vi "Clear-value-reference.vi"(8 "error in (no error)":errorcluster, 11 "Correct. params. ref.":refnum<data-value>) -> (0 "error out":errorcluster, 3 "Correct params out":refnum<class "CV-Correction.lvclass">)   [LabVIEW 2013, in "CameraVision.lvlib" / "CV-Correction.lvclass"]
uses:
  CV-Correction.lvclass
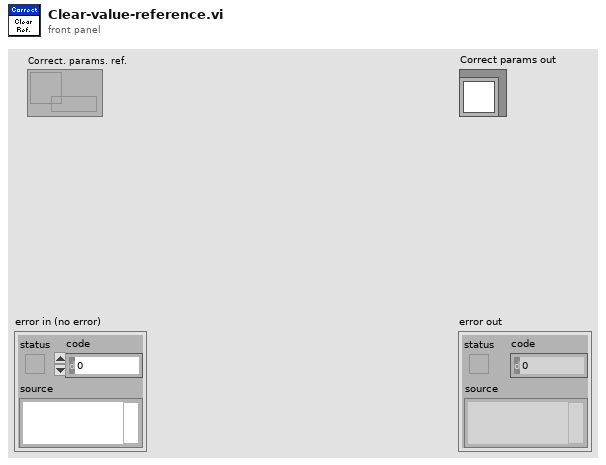
[diagram p1: front panel]
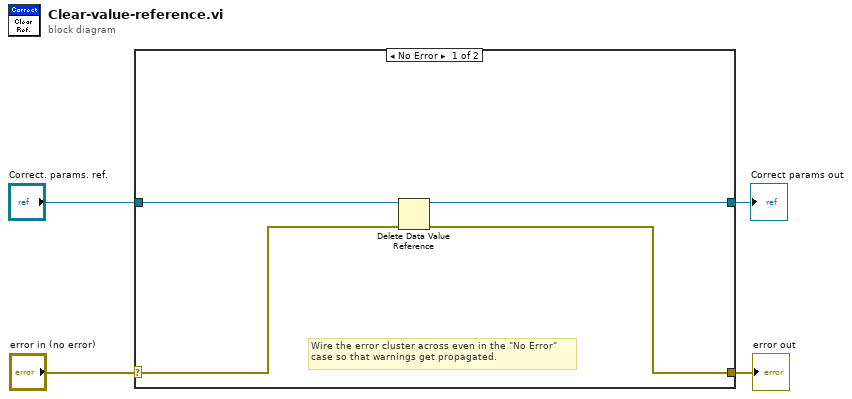
[diagram p0: block diagram]
diagram:
  n1 = case shown="No Error" "error in (no error)" {
    selector: "error in (no error)" -> [w7 w9]
    tunnel: [w6 w9] -> w3
    tunnel: [w5 _] -> w2
    tunnel: "Correct. params. ref." -> [w8 _]
    frame No Error {
      # "Wire the error cluster across even in the \"No Error\"\ncase so that warnings get propagated."
      n2 = Delete Data Value Reference(data value reference=w8, error in=w7) -> (data value=w5:refnum<class "CV-Correction.lvclass">, error out=w6:errorcluster)
    }
    frame Error {
    }
  }
  "error out" <- w3
  "Correct params out" <- w2
